vi "Set Bgnd Ref img UI from file-Boolean.vi"(8 "error in (no error)":errorcluster, 9 "Keys setup.Boolean":T2, 10 "Section name":string, 11 "User profile ini file ref":T1) -> (0 "error out":errorcluster, 3 "User profile ini file ref":T1)   [LabVIEW 2017]
uses:
  Typedefs/Ini file interface (Boolean).ctl
  <vilib>/Utility/config.llb/Config Data RefNum.ctl
  User Interface/Globals/gl_Windows Ctrl refs.vi
  <vilib>/Utility/config.llb/NI_LVConfig.lvlib
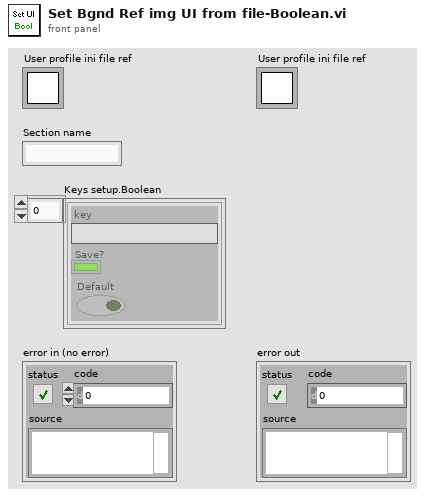
[diagram p1: front panel]
types:
  T1 = typedef "NI_LVConfig.lvlib/Config Data RefNum.ctl" = refnum<k1>
  T2 = typedef "Ini file interface (Boolean).ctl" = cluster{"key":string, "Save?":bool, "Default":bool}[]
  T3 = typedef "Live window-ctrl refs.ctl" = cluster{"This VI":refnum<vi>, "Pane":refnum<vi>, "Show REF Image Left":refnum<vi>, "Show REF Image Right":refnum<vi>, "Snapshot":refnum<vi>, "Left Image Palette":refnum<vi>, "Right Image Palette":refnum<vi>, "Left Channel":refnum<vi>, "Right Channel":refnum<vi>, "Left image intensity":refnum<vi>, "Right image intensity":refnum<vi>, "Left Image Display":T4, "Right Image Display":T4, "Refresh rate ind (Hz)":refnum<vi>, "Acq rate ind (Hz)":refnum<vi>, "Stop (ind)":refnum<vi>}
  T4 = typedef "Image display ref.ctl" = refnum<vi>
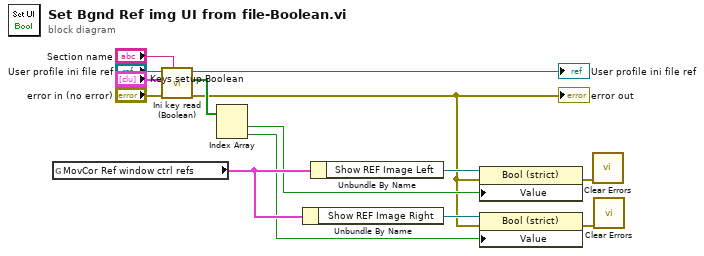
[diagram p0: block diagram]
diagram:
  n1 = global read "gl_Windows Ctrl refs.vi" "MovCor Ref window ctrl refs"() -> (w6:T3)
  n2 = call "Ini key read (Boolean).vi"("Section"="Section name", "error in (no error)"="error in (no error)", "Parameter names & setup"="Keys setup.Boolean", "Ini file refnum in"="User profile ini file ref") -> ("error out"=w3:errorcluster, "Value read/used"=w14:bool[], "Ini file refnum out"=→"User profile ini file ref":T1)  [unwired: 5 in]
  "error out" <- w3
  n3 = Index Array(array=w14) -> (element #1=w5:bool, element #2=w4:bool)  [unwired: 2 in]
  n4 = Unbundle By Name(w6) -> ("Show REF Image Right"=w8:refnum<vi>)
  n5 = Unbundle By Name(w6) -> ("Show REF Image Left"=w7:refnum<vi>)
  n6 = property class="Bool (strict)"(reference=w7, error in=w3, "Value"=w5) -> (error out=w2:errorcluster)  [unwired: 1 out]
  n7 = property class="Bool (strict)"(reference=w8, error in=w3, "Value"=w4) -> (error out=w1:errorcluster)  [unwired: 1 out]
  n8 = call <vilib>:"Clear Errors.vi"("error in (no error)"=w2) -> ()  [unwired: 5 in, 2 out]
  n9 = call <vilib>:"Clear Errors.vi"("error in (no error)"=w1) -> ()  [unwired: 5 in, 2 out]
